vi "Unit Test.vi"() -> ()   [LabVIEW 2019, in "Image.lvlib"]
uses:
  Image.lvlib
  LED/SubVI/Image Para.ctl
  MiControl-E/LV Source/ImageSystem/Cradle Zyla_1117/Ctl/seletion.ctl
  User Event/Controls/UE Abort Action.ctl
  Camera/Andor/Andor.lvlib
  Laser/Coherent/Coherent.lvlib
  LED/LED.lvlib
  Motion/Allmotion/Allmotion.lvlib
panel:
  out "Match Score":dbl
  in  "Match Pattern":bool
  in  "Image Para":T1[](array[typedef]) {"set shutter(s)" min=0.001 max=10.0 step=0.001; "Power(Amp)" min=15 max=100}
  in  "Align Laser":bool
  in  "Start Offset":i32
  out "LED Setup":string[][](array[string])=[["Light", "Cube"], ["UV", "2"], ["Red", "3"], ["Green", "4"], ["Blue-Red", "7"], ["Blue", "5"], ["UV-IR", "8"], ["UV-Red", "6"], ["BF", "6"]]
  in  "Focus Search":bool
  in  "Acquire Iamge":bool
  in  "Grab":bool
  out "Motion":bool
  out "LED":bool
  out "Laser":bool
  out "Camera":bool
  in  "Open":bool
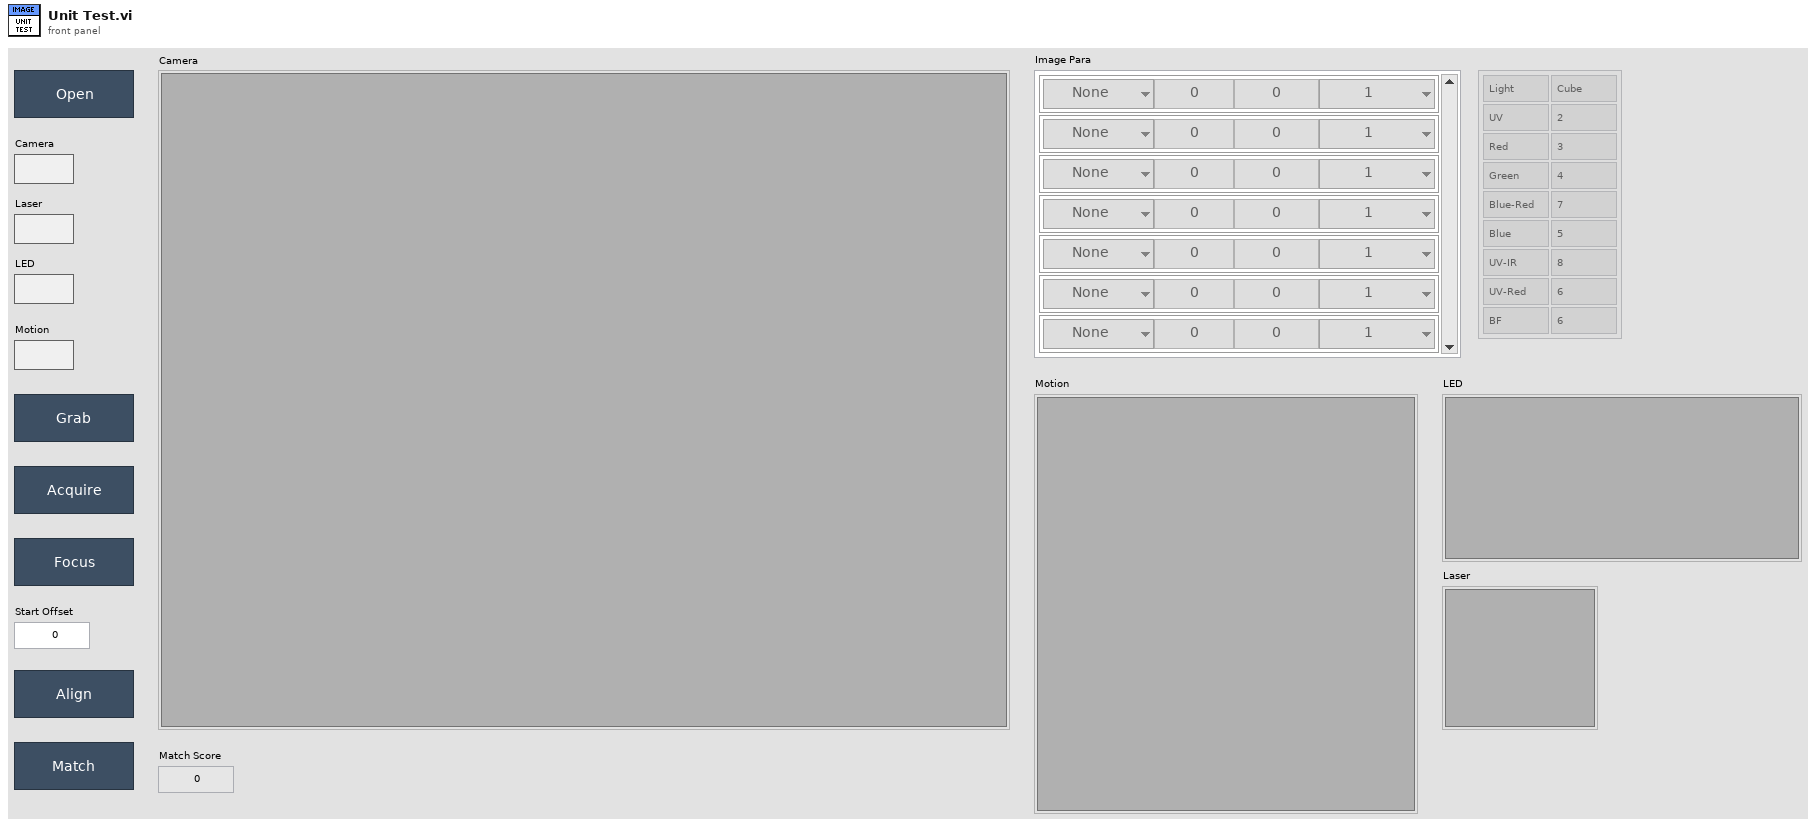
[diagram p1: front panel]
types:
  T1 = typedef "LED.lvlib/Image Para.ctl" = cluster{"Marker":T2, "Power(Amp)":u8, "set shutter(s)":dbl, "Cube":enum16{"1", "2", "3", "4", "5", "6", "7", "8"}}
  T2 = typedef "seletion.ctl" = enum16{"None", "Red", "Green", "Blue", "UV", "Green Laser", "Blue-Red", "UV-Red", "BF", "UV-IR"}
  T3 = typedef "UE Abort Action.ctl" = enum16{"Create", "Get", "Destroy"}
  T4 = typedef "ROI Descriptor" = cluster{"Global Rectangle":i32[], "Contours":cluster{"ID":enum32{"External", "Internal"}, "Type":u32, "Coordinates":i32[]}[]}
  T5 = cluster{"Image Path":path, "Start Offset":i32, "Template Path":path, "Disable Fine Search":bool, "ROI":T4}
  T6 = typedef "Andor.lvlib/SEQ Data.ctl" = cluster{"Initialize Sucess?":bool, "Image Ref":T7, "VI Refnum":refnum<vi>}
  T7 = typedef "IMAQ Image.ctl" = refnum<image>
  T8 = typedef "Coherent.lvlib/SEQ Data.ctl" = cluster{"Initialize Success?":bool, "VI Refnum":refnum<vi>}
  T9 = typedef "LED.lvlib/SEQ Data.ctl" = cluster{"Initialize Sucess?":bool, "BL2 Regulator":dbl, "BL1 Regulator":dbl, "Blood Sensor 1":dbl, "Blood Sensor 2":dbl, "Air Pressure Sensor":dbl, "Force Snesor 1":u32, "Force Snesor 2":u32, "VI Refnum":refnum<vi>}
  T10 = typedef "Allmotion.lvlib/SEQ Data.ctl" = cluster{"Position":i32[], "Arrived?":bool, "VISA name":refnum<visa-resource-name>, "Initialize Done?":bool, "State":string, "VI Refnum":refnum<vi>, "Dichroic Position":string[]}
  T11 = typedef "Image.lvlib/SEQ Data.ctl" = cluster{"Acquire Done?":bool, "Focus Done?":bool, "Align Done?":bool, "No Position Match?":bool, "Best Wheel Position":string, "Match Done?":bool, "Match Score":dbl, "Focus Score":dbl, "Match Position":cluster{"x":sgl, "y":sgl}}
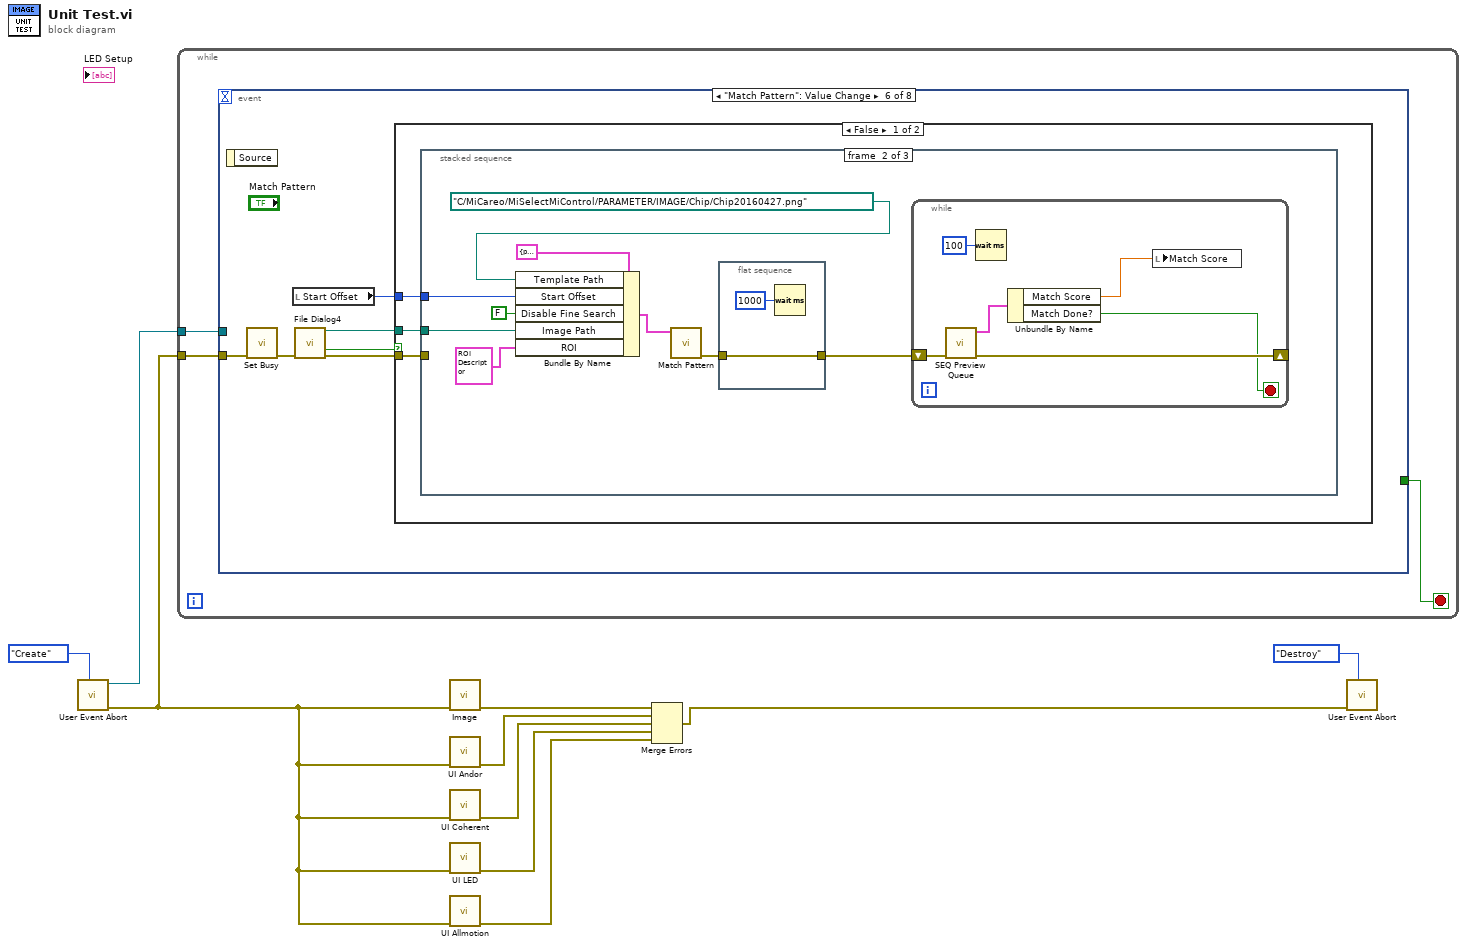
[diagram p0: block diagram]
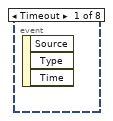
[diagram p2: hidden frame]
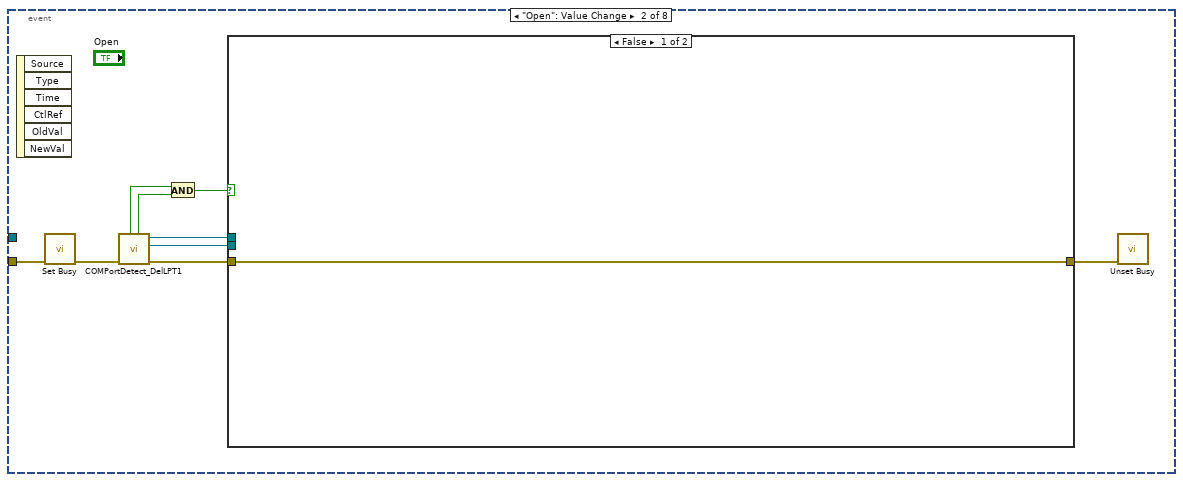
[diagram p3: hidden frame]
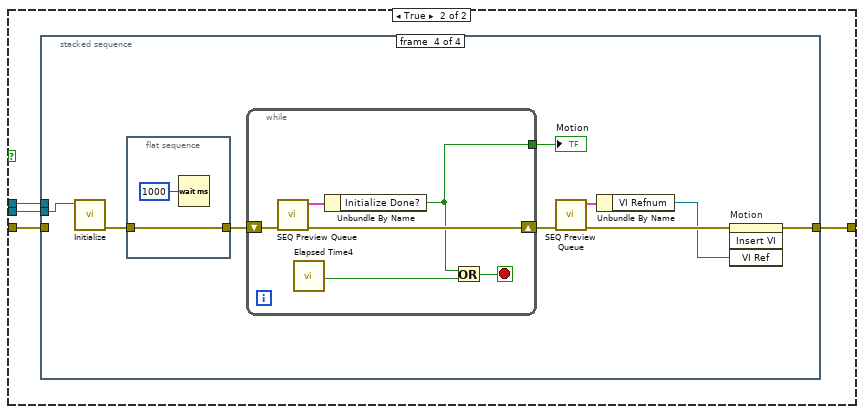
[diagram p4: hidden frame]
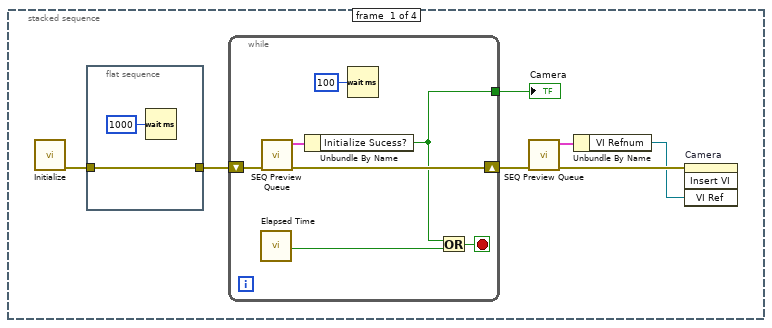
[diagram p5: hidden frame]
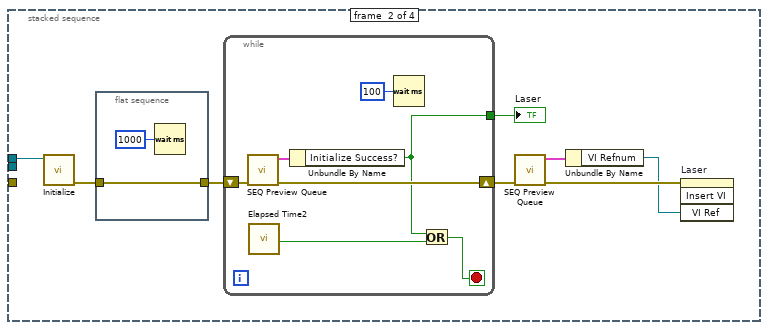
[diagram p6: hidden frame]
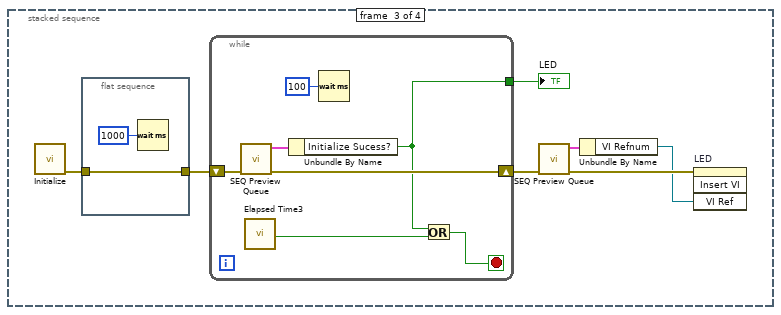
[diagram p7: hidden frame]
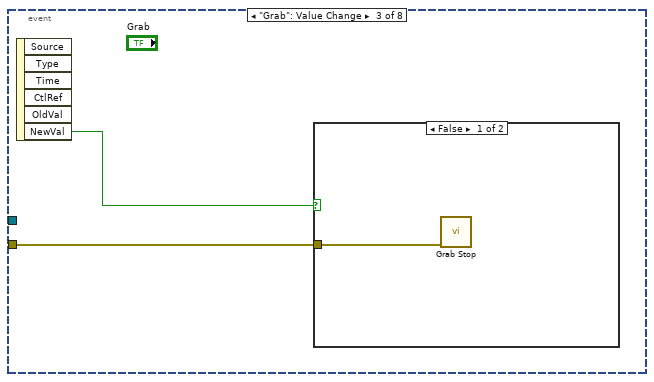
[diagram p8: hidden frame]
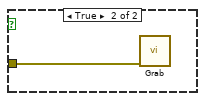
[diagram p9: hidden frame]
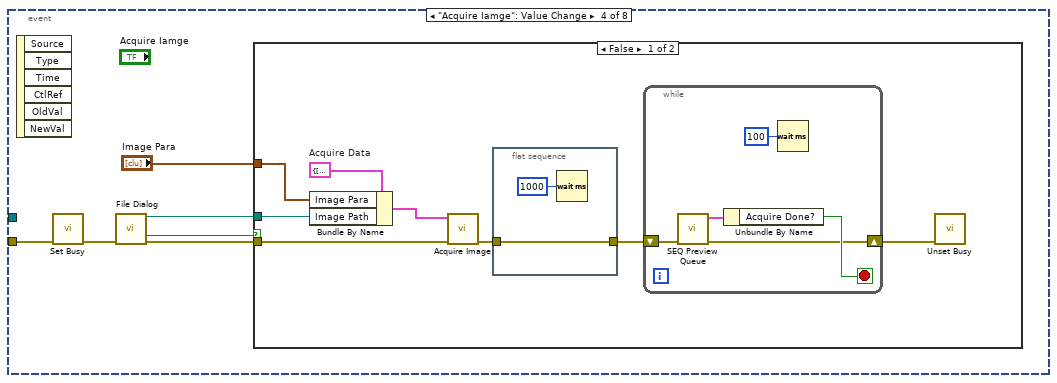
[diagram p10: hidden frame]
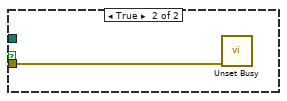
[diagram p11: hidden frame]
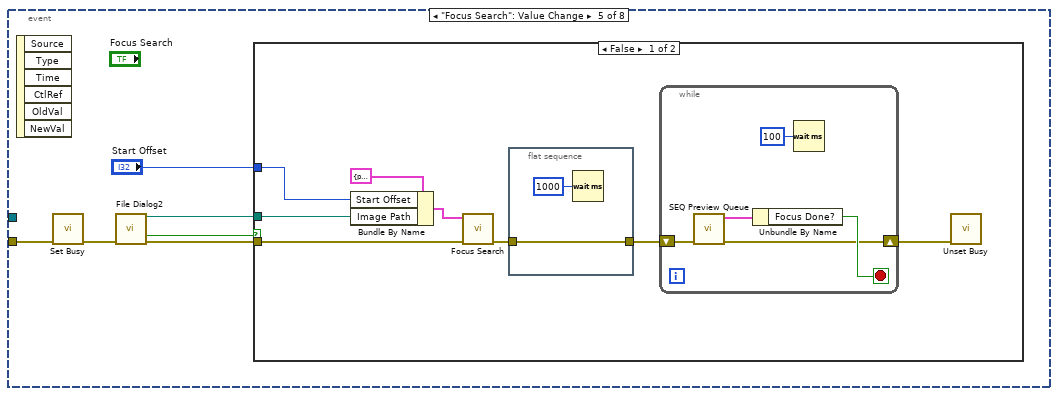
[diagram p12: hidden frame]
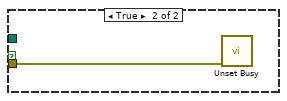
[diagram p13: hidden frame]
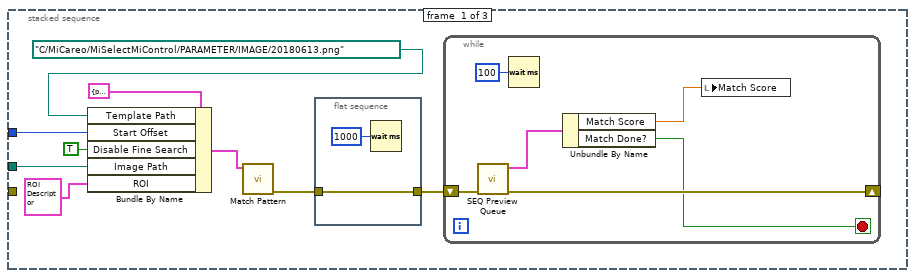
[diagram p14: hidden frame]
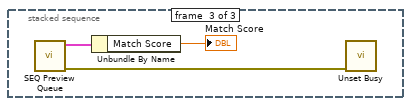
[diagram p15: hidden frame]
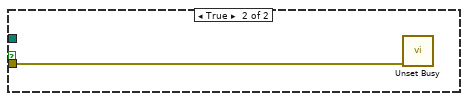
[diagram p16: hidden frame]
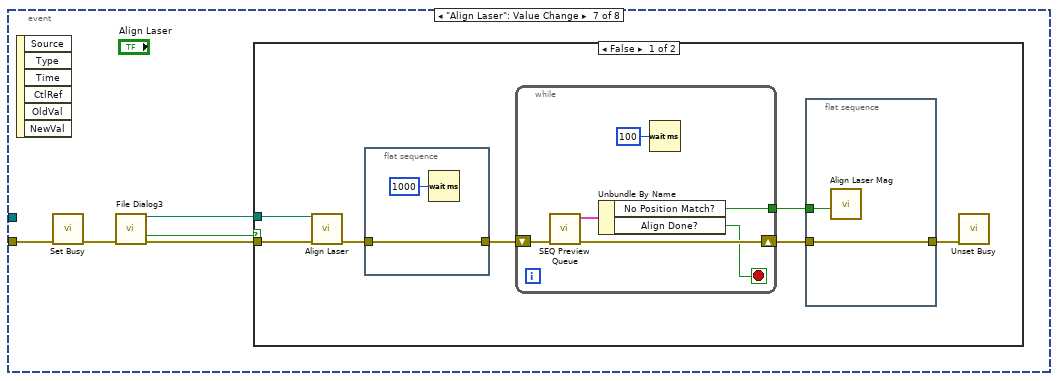
[diagram p17: hidden frame]
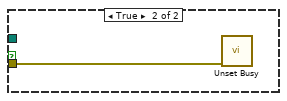
[diagram p18: hidden frame]
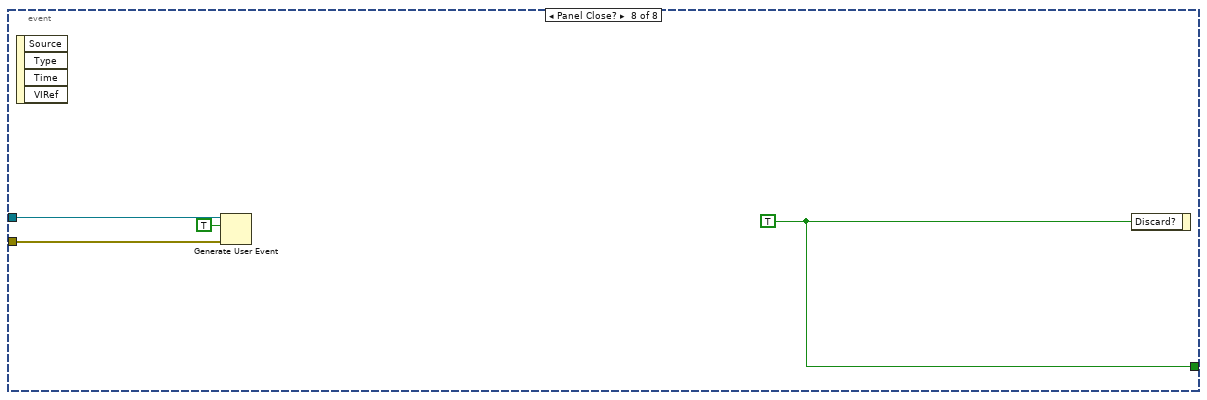
[diagram p19: hidden frame]
diagram:
  n1 = call "User Event Abort.vi"("Action"=UE_Abort_Action."Create") -> ("Error Out"=w1:errorcluster, "User Event Out"=w2:refnum<user-event>)  [unwired: 9 in]
  n2 = while {
    tunnel: w2 -> [w13]
    tunnel: w1 -> [w11]
    stop <- w12 stop-if-true
    n3 = event shown="[5] \"Match Pattern\": Value Change" {
      selector: _ -> [_ _ _ _ _ _ _ _]
      dyn-events: _ -> [_ _ _ _ _ _ _ _]
      timeout: _ -> [_ _ _ _ _ _ _ _]
      tunnel: w13 -> [_ _ _ _ _ _ _ w214]
      tunnel: [_ _ _ _ _ _ _ w215] -> w12
      tunnel: w11 -> [_ w22 w95 w100 w122 w144 w190 w213]
      event Timeout {
        n4 = event-data() -> ()  [unwired: 1 in, 3 out]
      }
      event "Open": Value Change {
        n5 = event-data() -> ()  [unwired: 1 in, 6 out]
        n6 = call <vilib>:"Set Busy.vi"("error in (no error)"=w22) -> ("error out"=w20:errorcluster)  [unwired: 9 in, 1 out]
        n7 = call "COMPortDetect_DelLPT1.vi"("error in"=w20) -> ("error out"=w19:errorcluster, "VISA motion"=w14:refnum<visa-resource-name>, "VISA laser"=w15:refnum<visa-resource-name>, "Motion Find?"=w17:bool, "Laser Find?"=w18:bool)  [unwired: 6 in]
        n8 = And(x=w18, y=w17) -> (x .and. y?=w16:bool)
        n9 = case shown="False" w16 {
          tunnel: w19 -> [w23 w27]
          tunnel: [w23 w26] -> w21
          tunnel: w15 -> [_ w25]
          tunnel: w14 -> [_ w24]
          frame False {
          }
          frame True {
            n10 = stacked-sequence {
              tunnel: w27 -> [_ _ _ _]
              tunnel: [_ _ _ w78] -> w26
              tunnel: w25 -> [_ w44 _ _]
              tunnel: w24 -> [_ _ _ w77]
              frame #0 {
                n11 = call "Initialize.vi"() -> ("Error Out"=w34:errorcluster)  [unwired: 11 in]
                n12 = flat-sequence {
                  tunnel: w34 -> [w42]
                  tunnel: [w42] -> w33
                  frame #0 {
                    n13 = Wait (ms)(milliseconds to wait=u32 1000) -> ()  [unwired: 1 out]
                  }
                }
                n14 = while {
                  shift-right: [w36] -> w32
                  shift-left: w33 -> [w40]
                  tunnel: [w35] -> w28
                  stop <- w38 stop-if-true
                  n15 = call "Elapsed Time"() -> ("Time has Elapsed"=w37:bool)  [unwired: 12 in, 7 out]
                  n16 = call "SEQ Preview Queue.vi"("error in"=w40) -> ("error out"=w36:errorcluster, "SEQ Data"=w39:T6)  [unwired: 9 in]
                  n17 = Unbundle By Name(w39) -> ("Initialize Sucess?"=w35:bool)
                  n18 = Wait (ms)(milliseconds to wait=u32 100) -> ()  [unwired: 1 out]
                  n19 = Or(x=w35, y=w37) -> (x .or. y?=w38:bool)
                }
                "Camera" <- w28
                n20 = call "SEQ Preview Queue.vi"("error in"=w32) -> ("error out"=w31:errorcluster, "SEQ Data"=w30:T6)  [unwired: 9 in]
                n21 = Unbundle By Name(w30) -> ("VI Refnum"=w29:refnum<vi>)
                n22 = invoke on="Camera" class="SubPnl" method="Insert VI"(error in=w31, "VI Ref"=w29) -> ()  [unwired: 2 in, 4 out]
              }
              frame #1 {
                n23 = call "Initialize.vi"("VISA in"=w44) -> ("Error Out"=w51:errorcluster)  [unwired: 10 in]
                n24 = flat-sequence {
                  tunnel: w51 -> [w59]
                  tunnel: [w59] -> w50
                  frame #0 {
                    n25 = Wait (ms)(milliseconds to wait=u32 1000) -> ()  [unwired: 1 out]
                  }
                }
                n26 = while {
                  shift-right: [w53] -> w49
                  shift-left: w50 -> [w58]
                  tunnel: [w52] -> w48
                  stop <- w54 stop-if-true
                  n27 = call "SEQ Preview Queue.vi"("error in"=w58) -> ("error out"=w53:errorcluster, "SEQ Data"=w57:T8)  [unwired: 9 in]
                  n28 = call "Elapsed Time2"() -> ("Time has Elapsed"=w55:bool)  [unwired: 12 in, 7 out]
                  n29 = Unbundle By Name(w57) -> ("Initialize Success?"=w52:bool)
                  n30 = Wait (ms)(milliseconds to wait=u32 100) -> ()  [unwired: 1 out]
                  n31 = Or(x=w52, y=w55) -> (x .or. y?=w54:bool)
                }
                "Laser" <- w48
                n32 = call "SEQ Preview Queue.vi"("error in"=w49) -> ("error out"=w46:errorcluster, "SEQ Data"=w47:T8)  [unwired: 9 in]
                n33 = Unbundle By Name(w47) -> ("VI Refnum"=w45:refnum<vi>)
                n34 = invoke on="Laser" class="SubPnl" method="Insert VI"(error in=w46, "VI Ref"=w45) -> ()  [unwired: 2 in, 4 out]
              }
              frame #2 {
                n35 = call "Initialize.vi"() -> ("Error Out"=w67:errorcluster)  [unwired: 11 in]
                n36 = flat-sequence {
                  tunnel: w67 -> [w75]
                  tunnel: [w75] -> w66
                  frame #0 {
                    n37 = Wait (ms)(milliseconds to wait=u32 1000) -> ()  [unwired: 1 out]
                  }
                }
                n38 = while {
                  shift-right: [w72] -> w65
                  shift-left: w66 -> [w74]
                  tunnel: [w68] -> w64
                  stop <- w69 stop-if-true
                  n39 = call "SEQ Preview Queue.vi"("error in"=w74) -> ("error out"=w72:errorcluster, "SEQ Data"=w71:T9)  [unwired: 9 in]
                  n40 = call "Elapsed Time3"() -> ("Time has Elapsed"=w70:bool)  [unwired: 12 in, 7 out]
                  n41 = Unbundle By Name(w71) -> ("Initialize Sucess?"=w68:bool)
                  n42 = Wait (ms)(milliseconds to wait=u32 100) -> ()  [unwired: 1 out]
                  n43 = Or(x=w68, y=w70) -> (x .or. y?=w69:bool)
                }
                "LED" <- w64
                n44 = call "SEQ Preview Queue.vi"("error in"=w65) -> ("error out"=w62:errorcluster, "SEQ Data"=w63:T9)  [unwired: 9 in]
                n45 = Unbundle By Name(w63) -> ("VI Refnum"=w61:refnum<vi>)
                n46 = invoke on="LED" class="SubPnl" method="Insert VI"(error in=w62, "VI Ref"=w61) -> ()  [unwired: 2 in, 4 out]
              }
              frame #3 {
                n47 = call "Initialize.vi"("VISA in"=w77) -> ("Error Out"=w85:errorcluster)  [unwired: 10 in]
                n48 = flat-sequence {
                  tunnel: w85 -> [w86]
                  tunnel: [w86] -> w84
                  frame #0 {
                    n49 = Wait (ms)(milliseconds to wait=u32 1000) -> ()  [unwired: 1 out]
                  }
                }
                n50 = while {
                  shift-right: [w90] -> w83
                  shift-left: w84 -> [w93]
                  tunnel: [w88] -> w81
                  stop <- w91 stop-if-true
                  n51 = call "SEQ Preview Queue.vi"("error in"=w93) -> ("error out"=w90:errorcluster, "SEQ Data"=w92:T10)  [unwired: 9 in]
                  n52 = call "Elapsed Time4"() -> ("Time has Elapsed"=w89:bool)  [unwired: 12 in, 7 out]
                  n53 = Unbundle By Name(w92) -> ("Initialize Done?"=w88:bool)
                  n54 = Or(x=w88, y=w89) -> (x .or. y?=w91:bool)
                }
                "Motion" <- w81
                n55 = call "SEQ Preview Queue.vi"("error in"=w83) -> ("error out"=w80:errorcluster, "SEQ Data"=w82:T10)  [unwired: 9 in]
                n56 = Unbundle By Name(w82) -> ("VI Refnum"=w79:refnum<vi>)
                n57 = invoke on="Motion" class="SubPnl" method="Insert VI"(error in=w80, "VI Ref"=w79) -> (error out=w78:errorcluster)  [unwired: 2 in, 3 out]
              }
            }
          }
        }
        n58 = call <vilib>:"Unset Busy.vi"("error in (no error)"=w21) -> ()  [unwired: 10 in, 1 out]
      }
      event "Grab": Value Change {
        n59 = event-data() -> ("NewVal"=w94:bool)  [unwired: 1 in, 5 out]
        n60 = case shown="False" w94 {
          tunnel: w95 -> [w96 w97]
          frame False {
            n61 = call "Grab Stop.vi"("Error In"=w96) -> ()  [unwired: 10 in, 1 out]
          }
          frame True {
            n62 = call "Grab.vi"("Error In"=w97) -> ()  [unwired: 10 in, 1 out]
          }
        }
      }
      event "Acquire Iamge": Value Change {
        n63 = event-data() -> ()  [unwired: 1 in, 6 out]
        n64 = call <vilib>:"Set Busy.vi"("error in (no error)"=w100) -> ("error out"=w99:errorcluster)  [unwired: 9 in, 1 out]
        n65 = call "File Dialog"("error in"=w99) -> ("selected path"=w102:path, "cancelled"=w103:bool, "error out"=w101:errorcluster)  [unwired: 11 in, 1 out]
        n66 = case shown="False" w103 {
          tunnel: w102 -> [w106 _]
          tunnel: w101 -> [w109 w119]
          tunnel: "Image Para" -> [w104 _]
          frame False {
            w107 = cluster{"Image Para":T1[], "Image Path":path} {"Image Para"=[], "Image Path"=path ""}  # Acquire Data
            n67 = Bundle By Name(cluster=w107, "Image Para"=w104, "Image Path"=w106) -> (w105:cluster{"Image Para":T1[], "Image Path":path})
            n68 = call "Acquire Image.vi"("Error In"=w109, "Acquire Data"=w105) -> ("Error Out"=w108:errorcluster)  [unwired: 9 in]
            n69 = flat-sequence {
              tunnel: w108 -> [w117]
              tunnel: [w117] -> w111
              frame #0 {
                n70 = Wait (ms)(milliseconds to wait=u32 1000) -> ()  [unwired: 1 out]
              }
            }
            n71 = while {
              shift-right: [w112] -> w110
              shift-left: w111 -> [w116]
              stop <- w113 stop-if-true
              n72 = call "SEQ Preview Queue.vi"("error in"=w116) -> ("error out"=w112:errorcluster, "SEQ Data"=w114:T11)  [unwired: 9 in]
              n73 = Unbundle By Name(w114) -> ("Acquire Done?"=w113:bool)
              n74 = Wait (ms)(milliseconds to wait=u32 100) -> ()  [unwired: 1 out]
            }
            n75 = call <vilib>:"Unset Busy.vi"("error in (no error)"=w110) -> ()  [unwired: 10 in, 1 out]
          }
          frame True {
            n76 = call <vilib>:"Unset Busy.vi"("error in (no error)"=w119) -> ()  [unwired: 10 in, 1 out]
          }
        }
      }
      event "Focus Search": Value Change {
        n77 = event-data() -> ()  [unwired: 1 in, 6 out]
        n78 = call <vilib>:"Set Busy.vi"("error in (no error)"=w122) -> ("error out"=w121:errorcluster)  [unwired: 9 in, 1 out]
        n79 = call "File Dialog2"("error in"=w121) -> ("selected path"=w124:path, "cancelled"=w125:bool, "error out"=w123:errorcluster)  [unwired: 11 in, 1 out]
        n80 = case shown="False" w125 {
          tunnel: w124 -> [w128 _]
          tunnel: w123 -> [w133 w141]
          tunnel: "Start Offset" -> [w126 _]
          frame False {
            n81 = Bundle By Name(cluster=cluster{"Image Path":path, "Start Offset":i32} {"Image Path"=path "", "Start Offset"=0} ("Focus Data"), "Start Offset"=w126, "Image Path"=w128) -> (w127:cluster{"Image Path":path, "Start Offset":i32})
            n82 = call "Focus Search.vi"("Error In"=w133, "Focus Data"=w127) -> ("Error Out"=w132:errorcluster)  [unwired: 9 in]
            n83 = flat-sequence {
              tunnel: w132 -> [w139]
              tunnel: [w139] -> w131
              frame #0 {
                n84 = Wait (ms)(milliseconds to wait=u32 1000) -> ()  [unwired: 1 out]
              }
            }
            n85 = while {
              shift-right: [w134] -> w130
              shift-left: w131 -> [w138]
              stop <- w135 stop-if-true
              n86 = call "SEQ Preview Queue.vi"("error in"=w138) -> ("error out"=w134:errorcluster, "SEQ Data"=w136:T11)  [unwired: 9 in]
              n87 = Unbundle By Name(w136) -> ("Focus Done?"=w135:bool)
              n88 = Wait (ms)(milliseconds to wait=u32 100) -> ()  [unwired: 1 out]
            }
            n89 = call <vilib>:"Unset Busy.vi"("error in (no error)"=w130) -> ()  [unwired: 10 in, 1 out]
          }
          frame True {
            n90 = call <vilib>:"Unset Busy.vi"("error in (no error)"=w141) -> ()  [unwired: 10 in, 1 out]
          }
        }
      }
      event "Match Pattern": Value Change {
        n91 = event-data() -> ()  [unwired: 1 in, 1 out]
        n92 = call <vilib>:"Set Busy.vi"("error in (no error)"=w144) -> ("error out"=w143:errorcluster)  [unwired: 9 in, 1 out]
        n93 = local read "Start Offset"() -> (w142:i32)
        n94 = call "File Dialog4"("error in"=w143) -> ("selected path"=w146:path, "cancelled"=w147:bool, "error out"=w145:errorcluster)  [unwired: 11 in, 1 out]
        n95 = case shown="False" w147 {
          tunnel: w146 -> [w149 _]
          tunnel: w145 -> [w150 w188]
          tunnel: w142 -> [w148 _]
          frame False {
            n96 = stacked-sequence {
              tunnel: w150 -> [_ _ _]
              tunnel: w149 -> [w157 w174 _]
              tunnel: w148 -> [w156 w173 _]
              frame #0 {
                n97 = Bundle By Name(cluster=T5 {"Image Path"=path "", "Start Offset"=0, "Template Path"=path "", "Disable Fine Search"=FALSE, "ROI"={"Global Rectangle"=[], "Contours"=[]}} ("Match Data"), "Template Path"=path "C:/MiCareo/MiSelectMiControl/PARAMETER/IMAGE/20180613.png" ("File Path"), "Start Offset"=w156, "Disable Fine Search"=TRUE, "Image Path"=w157, "ROI"=T4 {"Global Rectangle"=[0, 0, 2560, 2160], "Contours"=[{"ID"=enum."External", "Type"=3, "Coordinates"=[0, 0, 2560, 2160, 0]}]}) -> (w152:T5)
                n98 = call "Match Pattern.vi"("Match Data"=w152) -> ("Error Out"=w159:errorcluster)  [unwired: 10 in]
                n99 = flat-sequence {
                  tunnel: w159 -> [w166]
                  tunnel: [w166] -> w158
                  frame #0 {
                    n100 = Wait (ms)(milliseconds to wait=u32 1000) -> ()  [unwired: 1 out]
                  }
                }
                n101 = while {
                  shift-right: [w162] -> _
                  shift-left: w158 -> [w165]
                  stop <- w161 stop-if-true
                  n102 = call "SEQ Preview Queue.vi"("error in"=w165) -> ("error out"=w162:errorcluster, "SEQ Data"=w163:T11)  [unwired: 9 in]
                  n103 = Wait (ms)(milliseconds to wait=u32 100) -> ()  [unwired: 1 out]
                  n104 = Unbundle By Name(w163) -> ("Match Score"=w160:dbl, "Match Done?"=w161:bool)
                  n105 = local write "Match Score"(w160) -> ()
                }
              }
              frame #1 {
                n106 = Bundle By Name(cluster=T5 {"Image Path"=path "", "Start Offset"=0, "Template Path"=path "", "Disable Fine Search"=FALSE, "ROI"={"Global Rectangle"=[], "Contours"=[]}} ("Match Data"), "Template Path"=path "C:/MiCareo/MiSelectMiControl/PARAMETER/IMAGE/Chip/Chip20160427.png", "Start Offset"=w173, "Disable Fine Search"=FALSE, "Image Path"=w174, "ROI"=T4 {"Global Rectangle"=[1030, 830, 1530, 1330], "Contours"=[{"ID"=enum."External", "Type"=3, "Coordinates"=[1030, 830, 1530, 1330, 0]}]}) -> (w168:T5)
                n107 = call "Match Pattern.vi"("Match Data"=w168) -> ("Error Out"=w176:errorcluster)  [unwired: 10 in]
                n108 = flat-sequence {
                  tunnel: w176 -> [w183]
                  tunnel: [w183] -> w175
                  frame #0 {
                    n109 = Wait (ms)(milliseconds to wait=u32 1000) -> ()  [unwired: 1 out]
                  }
                }
                n110 = while {
                  shift-right: [w179] -> _
                  shift-left: w175 -> [w182]
                  stop <- w178 stop-if-true
                  n111 = call "SEQ Preview Queue.vi"("error in"=w182) -> ("error out"=w179:errorcluster, "SEQ Data"=w180:T11)  [unwired: 9 in]
                  n112 = Wait (ms)(milliseconds to wait=u32 100) -> ()  [unwired: 1 out]
                  n113 = Unbundle By Name(w180) -> ("Match Score"=w177:dbl, "Match Done?"=w178:bool)
                  n114 = local write "Match Score"(w177) -> ()
                }
              }
              frame #2 {
                n115 = call "SEQ Preview Queue.vi"() -> ("error out"=w186:errorcluster, "SEQ Data"=w187:T11)  [unwired: 10 in]
                n116 = Unbundle By Name(w187) -> ("Match Score"=→"Match Score":dbl)
                n117 = call <vilib>:"Unset Busy.vi"("error in (no error)"=w186) -> ()  [unwired: 10 in, 1 out]
              }
            }
          }
          frame True {
            n118 = call <vilib>:"Unset Busy.vi"("error in (no error)"=w188) -> ()  [unwired: 10 in, 1 out]
          }
        }
      }
      event "Align Laser": Value Change {
        n119 = event-data() -> ()  [unwired: 1 in, 6 out]
        n120 = call <vilib>:"Set Busy.vi"("error in (no error)"=w190) -> ("error out"=w189:errorcluster)  [unwired: 9 in, 1 out]
        n121 = call "File Dialog3"("error in"=w189) -> ("selected path"=w192:path, "cancelled"=w193:bool, "error out"=w191:errorcluster)  [unwired: 11 in, 1 out]
        n122 = case shown="False" w193 {
          tunnel: w192 -> [w197 _]
          tunnel: w191 -> [w200 w211]
          frame False {
            n123 = call "Align Laser.vi"("Error In"=w200, "Image Path"=w197) -> ("Error Out"=w199:errorcluster)  [unwired: 9 in]
            n124 = flat-sequence {
              tunnel: w199 -> [w209]
              tunnel: [w209] -> w198
              frame #0 {
                n125 = Wait (ms)(milliseconds to wait=u32 1000) -> ()  [unwired: 1 out]
              }
            }
            n126 = while {
              shift-right: [w205] -> w195
              shift-left: w198 -> [w208]
              tunnel: [w203] -> w196
              stop <- w204 stop-if-true
              n127 = call "SEQ Preview Queue.vi"("error in"=w208) -> ("error out"=w205:errorcluster, "SEQ Data"=w206:T11)  [unwired: 9 in]
              n128 = Unbundle By Name(w206) -> ("No Position Match?"=w203:bool, "Align Done?"=w204:bool)
              n129 = Wait (ms)(milliseconds to wait=u32 100) -> ()  [unwired: 1 out]
            }
            n130 = flat-sequence {
              tunnel: w196 -> [w202]
              tunnel: w195 -> [w201]
              tunnel: [w201] -> w194
              frame #0 {
                n131 = call "Align Laser Mag"("Enable"=w202) -> ()  [unwired: 9 in, 2 out]
              }
            }
            n132 = call <vilib>:"Unset Busy.vi"("error in (no error)"=w194) -> ()  [unwired: 10 in, 1 out]
          }
          frame True {
            n133 = call <vilib>:"Unset Busy.vi"("error in (no error)"=w211) -> ()  [unwired: 10 in, 1 out]
          }
        }
      }
      event Panel Close? {
        w215 = TRUE ("Discard?")
        n134 = event-data() -> ()  [unwired: 1 in, 4 out]
        n135 = Generate User Event(user event=w214, event data cluster=TRUE ("event data"), error in=w213) -> ()  [unwired: 1 in, 2 out]
        n136 = event-data("Discard?"=w215) -> ()  [unwired: 1 in, 1 out]
      }
    }
  }
  n137 = call "Image.vi"("error in"=w1) -> ("error out"=w10:errorcluster)  [unwired: 10 in]
  n138 = call "UI Andor.vi"("error in"=w1) -> ("error out"=w9:errorcluster)  [unwired: 10 in]
  n139 = call "UI Coherent.vi"("error in"=w1) -> ("error out"=w8:errorcluster)  [unwired: 10 in]
  n140 = call "UI LED.vi"("error in"=w1) -> ("error out"=w7:errorcluster)  [unwired: 10 in]
  n141 = call "UI Allmotion.vi"("error in"=w1) -> ("error out"=w6:errorcluster)  [unwired: 10 in]
  n142 = Merge Errors(w10, w9, w8, w7, w6) -> (w5:errorcluster)
  n143 = call "User Event Abort.vi"("Action"=UE_Abort_Action."Destroy", "Error In"=w5) -> ()  [unwired: 8 in, 2 out]
